vi "Configuration Keys.vi"(8 "error in (no error)":errorcluster, 11 "Report in":refnum<class "Report.lvclass">) -> (0 "error out":errorcluster, 2 "Required Keys":string[](array[string]), 3 "Report out":refnum<class "Report.lvclass">)   [LabVIEW 2023, in "Report.lvlib" / "Report.lvclass"]
doc: "Configuration Keys is a dynamic dispatch VI that reads a full inheritance chain's required key list.\n\nThis means each instrument must override this vi, and call the parent method . The end result is a comprehensive list of required keys that must be present in an instrument's config.ini file to correctly function."
uses:
  Report.lvclass
  builds/Tools/Config.lvlibp/Config.lvclass
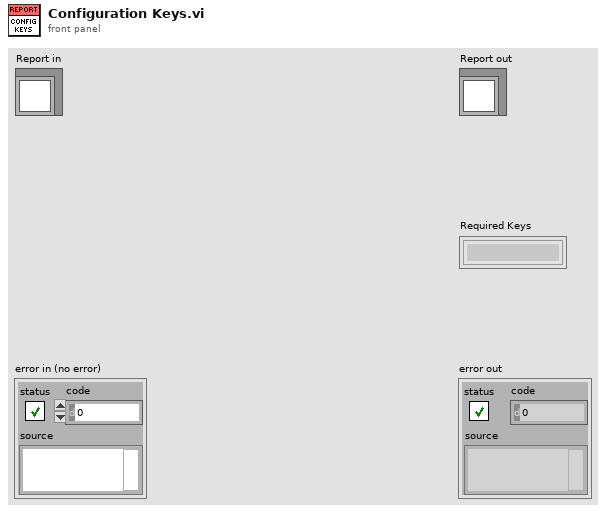
[diagram p1: front panel]
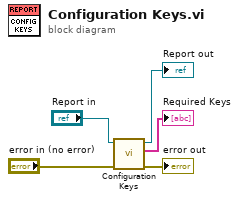
[diagram p0: block diagram]
diagram:
  n1 = call-parent "Configuration Keys.vi"("error in (no error)"="error in (no error)", "Config in"="Report in") -> ("error out"=→"error out":errorcluster, "Required Keys"=→"Required Keys":string[], "Config out"=→"Report out":refnum<class "Report.lvclass">)  [unwired: 7 in]
